vi "Set value by Variant.vi"(8 "error in (no error)":errorcluster, 10 "Variant":variant, 11 "Column in":refnum<class "Composed Column.lvclass">) -> (0 "error out":errorcluster, 3 "Column out":refnum<class "Composed Column.lvclass">)   [LabVIEW 2020, in "Composed Columns.lvlib" / "Composed Column.lvclass"]
uses:
  Composed Column.lvclass
  Composed Column.lvclass/Composed Column.ctl
  Composed Columns/Value Source Interface Class/Value Source.lvclass
  Value Type/Value Type.lvclass
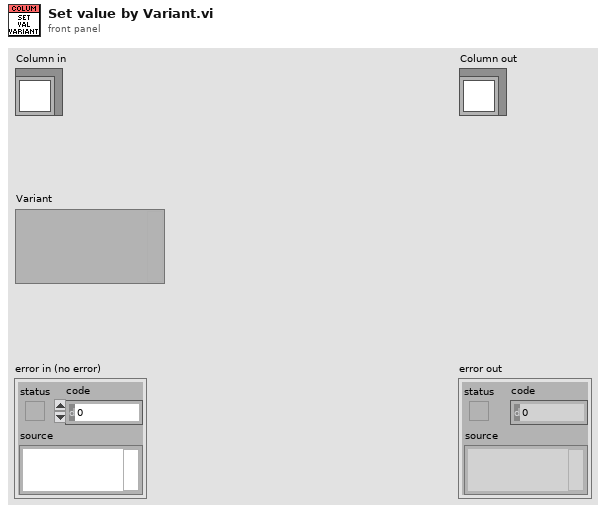
[diagram p1: front panel]
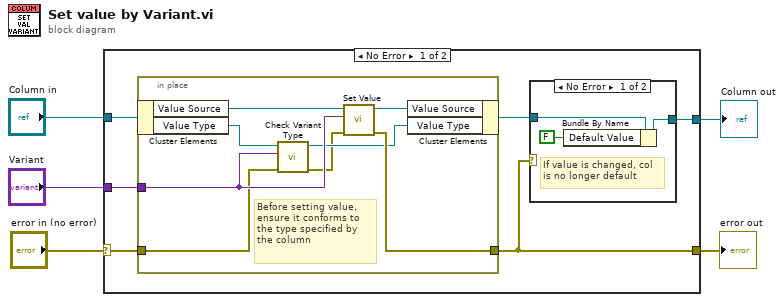
[diagram p0: block diagram]
diagram:
  n1 = case shown="No Error" "error in (no error)" {
    selector: "error in (no error)" -> [w10 w25]
    tunnel: [w7 w25] -> w2
    tunnel: "Column in" -> [w11 w24]
    tunnel: [w6 w24] -> w5
    tunnel: "Variant" -> [w9 _]
    frame No Error {
      n2 = in-place {
        in-place-border: w10 -> [w16]
        in-place-border: [w21] -> w7
        in-place-border: w9 -> [w20]
        # "Before setting value, ensure it conforms to the type specified by the column"
        n3 = in-place-cluster #1(w11) -> ("Value Source"=w23:refnum<class "Value Source.lvclass">, "Value Type"=w19:refnum<class "Value Type.lvclass">)
        n4 = call-dynamic "Check Variant Type.vi"("error in (no error)"=w16, "Variant"=w20, "Value Type in"=w19) -> ("error out"=w17:errorcluster, "Value Type out"=w18:refnum<class "Value Type.lvclass">)  [unwired: 7 in]
        n5 = call-dynamic "Set Value.vi"("error in (no error)"=w17, "Variant"=w20, "Value Source in"=w23) -> ("error out"=w21:errorcluster, "Value Source out"=w22:refnum<class "Value Source.lvclass">)  [unwired: 7 in]
        n6 = in-place-cluster #1("Value Source"=w22, "Value Type"=w18) -> (w8:refnum<class "Composed Column.lvclass">)
      }
      n7 = case shown="No Error" w7 {
        tunnel: w8 -> [w14 w15]
        tunnel: [w13 w15] -> w6
        frame No Error {
          # "If value is changed, col\nis no longer default"
          n8 = Bundle By Name(cluster=w14, "Default Value"=FALSE) -> (w13:refnum<class "Composed Column.lvclass">)
        }
        frame Error {
        }
      }
    }
    frame Error {
    }
  }
  "error out" <- w2
  "Column out" <- w5
